vi "SpeedCalculation.vi"(10 "Axis1":dbl, 11 "Axis2":dbl) -> (2 "Speed mm/s":dbl, 3 "Speed for card":dbl)   [LabVIEW 2017]
uses:
  Settings/Traverse-Settings-Global.vi
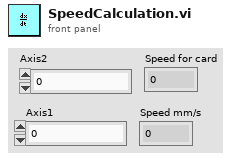
[diagram p1: front panel]
types:
  T1 = cluster{"Acceleration":dbl[], "Deceleration":dbl[], "Max Velocity":dbl[], "Speed":dbl, "Pulse/Degree":dbl, "Degre Factor":dbl[], "mm/rotation":dbl[]}
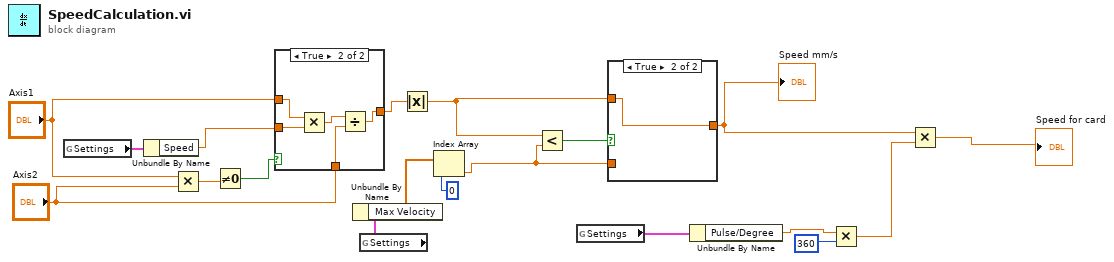
[diagram p0: block diagram]
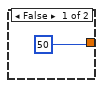
[diagram p2: hidden frame]
diagram:
  n1 = global read "Traverse-Settings-Global.vi" "Settings"() -> (w16:T1)
  n2 = Unbundle By Name(w16) -> ("Speed"=w7:dbl)
  n3 = Multiply(x="Axis1", y="Axis2") -> (x*y=w10:dbl)
  n4 = Not Equal To 0?(x=w10) -> (x != 0?=w11:bool)
  n5 = case shown="True" w11 {
    tunnel: "Axis2" -> [_ w23]
    tunnel: [50 w22] -> w18
    tunnel: "Axis1" -> [_ w21]
    tunnel: w7 -> [_ w25]
    frame False {
    }
    frame True {
      n6 = Multiply(x=w21, y=w25) -> (x*y=w24:dbl)
      n7 = Divide(x=w24, y=w23) -> (x/y=w22:dbl)
    }
  }
  n8 = global read "Traverse-Settings-Global.vi" "Settings"() -> (w15:T1)
  n9 = Unbundle By Name(w15) -> ("Max Velocity"=w12:dbl[])
  n10 = Absolute Value(x=w18) -> (abs(x)=w17:dbl)
  n11 = Index Array(array=w12, index=0) -> (element=w13:dbl)
  n12 = Less?(x=w17, y=w13) -> (x < y?=w19:bool)
  n13 = global read "Traverse-Settings-Global.vi" "Settings"() -> (w4:T1)
  n14 = case shown="True" w19 {
    tunnel: w17 -> [_ w27]
    tunnel: w13 -> [w26 _]
    tunnel: [w26 w27] -> w1
    frame False {
    }
    frame True {
    }
  }
  "Speed mm/s" <- w1
  n15 = Unbundle By Name(w4) -> ("Pulse/Degree"=w3:dbl)
  n16 = Multiply(x=w3, y=360) -> (x*y=w5:dbl)
  n17 = Multiply(x=w1, y=w5) -> (x*y=→"Speed for card":dbl)
